vi "1stAnd3rdorderFunc.FitFunc.vi"(3 "output control":T1, 4 "data":variant, 5 "X":dbl[](array[numeric]), 6 "Coefficients":dbl[](array[numeric])) -> (0 "error out":errorcluster, 1 "f'(X,a)":dbl[][](array[numeric]), 2 "f(X,a)":dbl[](array[numeric]))   [LabVIEW 2020, in "XYcenter.lvlib"]
uses:
  XYcenter.lvlib
  <vilib>/gmath/NumericalOptimization/LM_output select.ctl
  <vilib>/gmath/NI_Gmath.lvlib
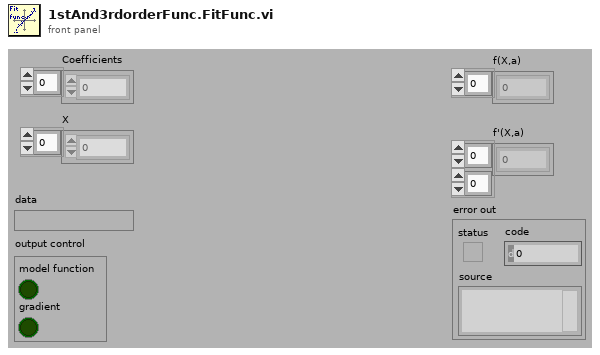
[diagram p1: front panel]
types:
  T1 = typedef "NI_Gmath.lvlib/LM_output select.ctl" = cluster{"model function":bool, "gradient":bool}
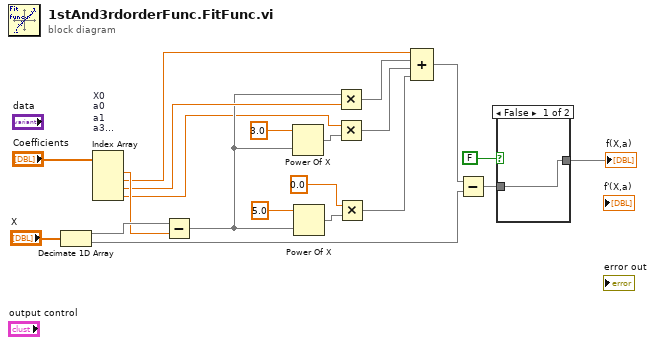
[diagram p0: block diagram]
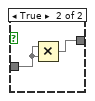
[diagram p2: hidden frame]
diagram:
  n1 = Decimate 1D Array("X") -> (w11:dbl[], w12:dbl[])
  n2 = Index Array "X0\na0\na1\na3\na5"(array="Coefficients") -> (element #1=w10:dbl, element #2=w9:dbl, element #3=w8:dbl, element #4=w4:dbl)  [unwired: 4 in]
  n3 = Subtract(x=w11, y=w10) -> (x-y=w5:dbl[])
  n4 = Power Of X(1:w5, 2:3.0) -> (0:w18:dbl[])
  n5 = Power Of X(1:w5, 2:5.0) -> (0:w6:dbl[])
  n6 = Multiply(x=w5, y=w8) -> (x*y=w17:dbl[])
  n7 = Multiply(x=w4, y=w18) -> (x*y=w13:dbl[])
  n8 = Multiply(x=0.0, y=w6) -> (x*y=w3:dbl[])
  n9 = Compound Arithmetic op=ADD(w9, w17, w13, w3) -> (w16:dbl[])
  n10 = Subtract(x=w16, y=w12) -> (x-y=w15:dbl[])
  n11 = case shown="False" FALSE {
    tunnel: w15 -> [w22 w24]
    tunnel: [w22 w23] -> w14
    frame False {
    }
    frame True {
      n12 = Multiply(x=w24, y=w24) -> (x*y=w23:dbl[])
    }
  }
  "f(X,a)" <- w14
